vi "DAQNaviGet_DIO_PortCount.vi"(8 "error in (no error)":errorcluster, 11 "task in":i32) -> (0 "error out":errorcluster, 2 "port count":i32, 3 "task out":i32)   [LabVIEW 2020]
uses:
  DAQNavi_LV.dll
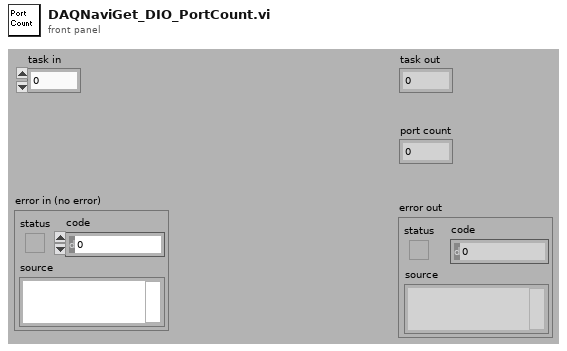
[diagram p1: front panel]
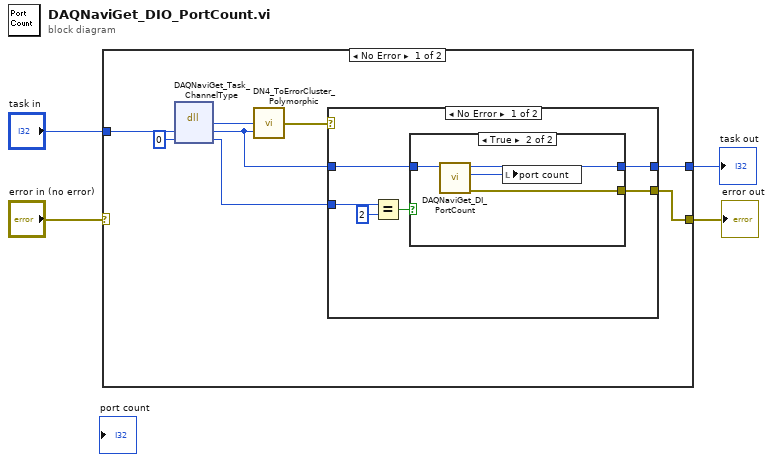
[diagram p0: block diagram]
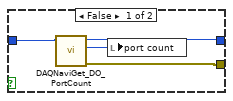
[diagram p2: hidden frame]
diagram:
  n1 = case shown="No Error" "error in (no error)" {
    selector: "error in (no error)" -> [_ w29]
    tunnel: "task in" -> [w12 w30]
    tunnel: [w7 w30] -> w2
    tunnel: [w6 w29] -> w1
    frame No Error {
      n2 = dll-call lib="DAQNavi_LV.dll" fn="DAQNaviGet_Task_ChannelType"("taskID"=w12, "type"=0) -> ("返回类型"=w10:i32, "taskID"=w8:i32, "type"=w5:i32)  [unwired: 3 in, 2 out]
      n3 = call "DN4_ToErrorCluster_Polymorphic.vi"("task id"=w8, "error code"=w10) -> ("error out"=w9:errorcluster)  [unwired: 3 out]
      n4 = case shown="No Error" w9 {
        selector: w9 -> [_ w27]
        tunnel: w8 -> [w16 w28]
        tunnel: [w15 w28] -> w7
        tunnel: [w14 w27] -> w6
        tunnel: w5 -> [w13 _]
        frame No Error {
          n5 = Equal?(x=w13, y=2) -> (x = y?=w17:bool)
          n6 = case shown="True" w17 {
            tunnel: w16 -> [w22 w26]
            tunnel: [w20 w24] -> w15
            tunnel: [w19 w23] -> w14
            frame False {
              n7 = call "DAQNaviGet_DO_PortCount.vi"("task in"=w22) -> ("error out"=w19:errorcluster, "port count"=w21:i32, "task out"=w20:i32)  [unwired: 1 in, 7 out]
              n8 = local write "port count"(w21) -> ()
            }
            frame True {
              n9 = call "DAQNaviGet_DI_PortCount.vi"("task in"=w26) -> ("error out"=w23:errorcluster, "port count"=w25:i32, "task out"=w24:i32)  [unwired: 1 in, 7 out]
              n10 = local write "port count"(w25) -> ()
            }
          }
        }
        frame Error {
        }
      }
    }
    frame Error {
    }
  }
  "task out" <- w2
  "error out" <- w1
